vi "Main.vi"(1 "重新开始？":bool) -> ()   [LabVIEW 2018]
panel:
  out "时间标识":timestamp format="%<%H:%M:%S\n%x>T"
  in  "参数设置":bool=TRUE
  in  "退出":bool
  in  "读取历史数据":bool=TRUE
  in  "保存数据":bool=TRUE
  in  "开始测量":bool=TRUE
  out "实时消息":T1
  # "任务选择"
  # "开始测量"
  # "退 出"
  # "保存数据"
  # "读取历史数据"
  # "功率"
  # "能量"
  # "时间"
  # "光谱"
  # "偏振"
  # "近远场"
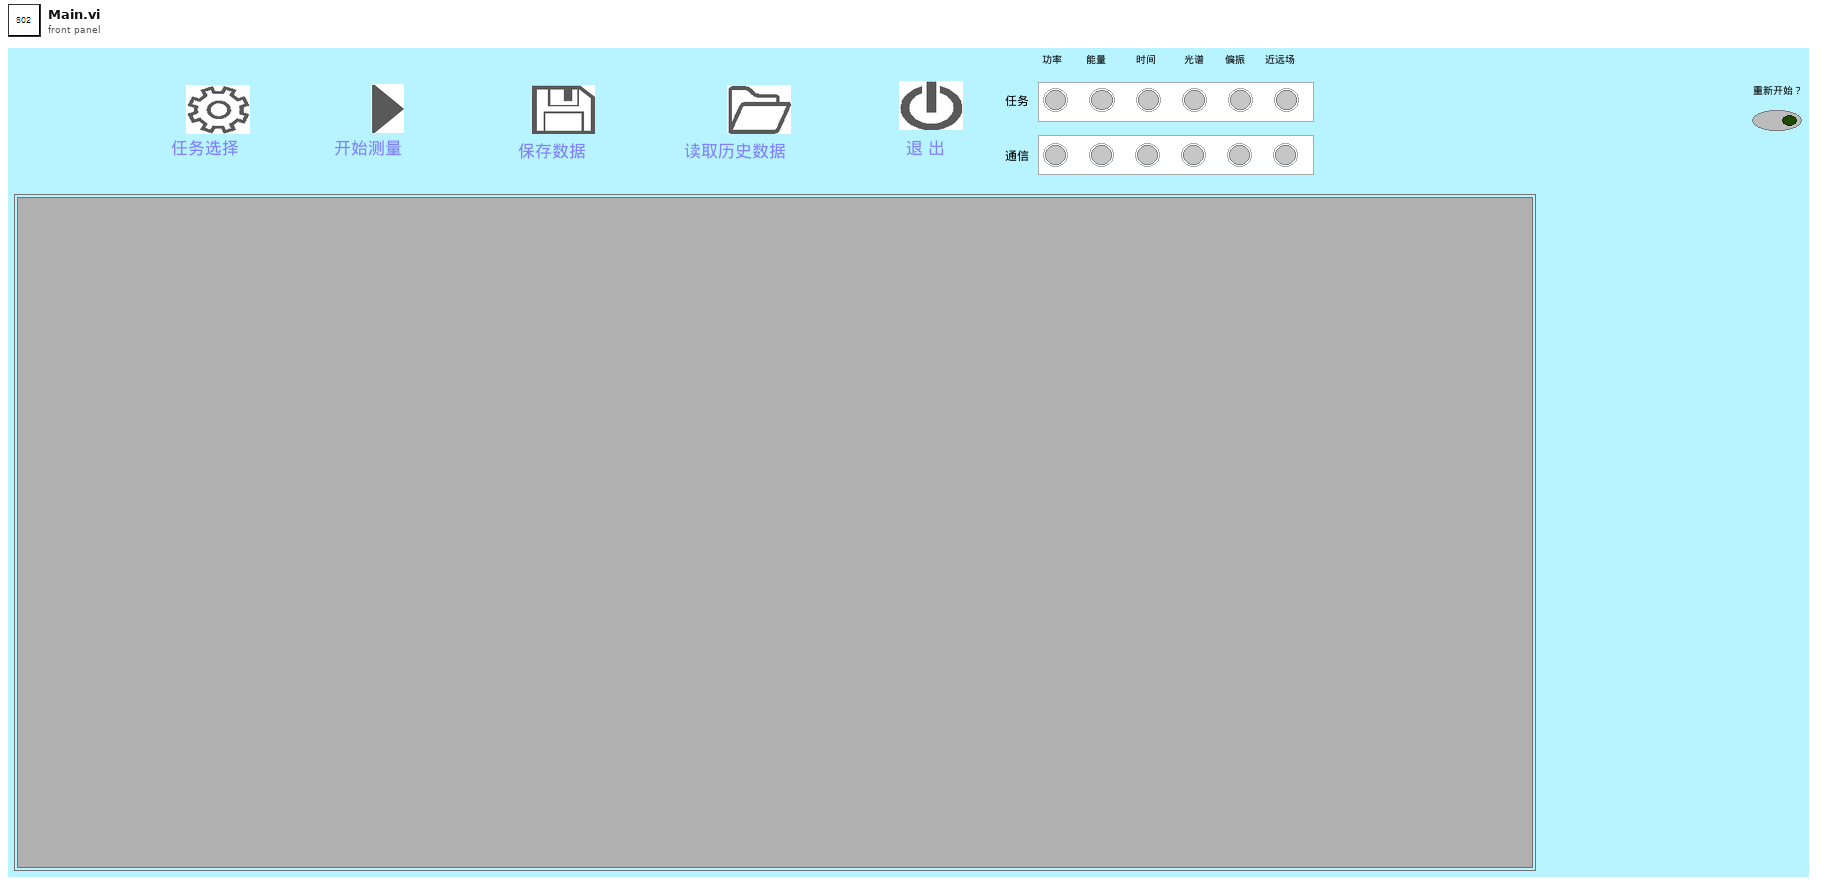
[diagram p1: front panel]
types:
  T1 = cluster{"任务":cluster{"功率任务":bool, "能量任务":bool, "时间波形任务":bool, "光谱任务":bool, "偏振任务":bool, "近远场任务":bool}, "通信":cluster{"功率通信":bool, "能量通信":bool, "时间波形通信":bool, "光谱通信":bool, "偏振通信":bool, "近远场通信":bool}}
  T2 = enum8{"Enabled", "Disabled", "Disabled and Grayed Out"}
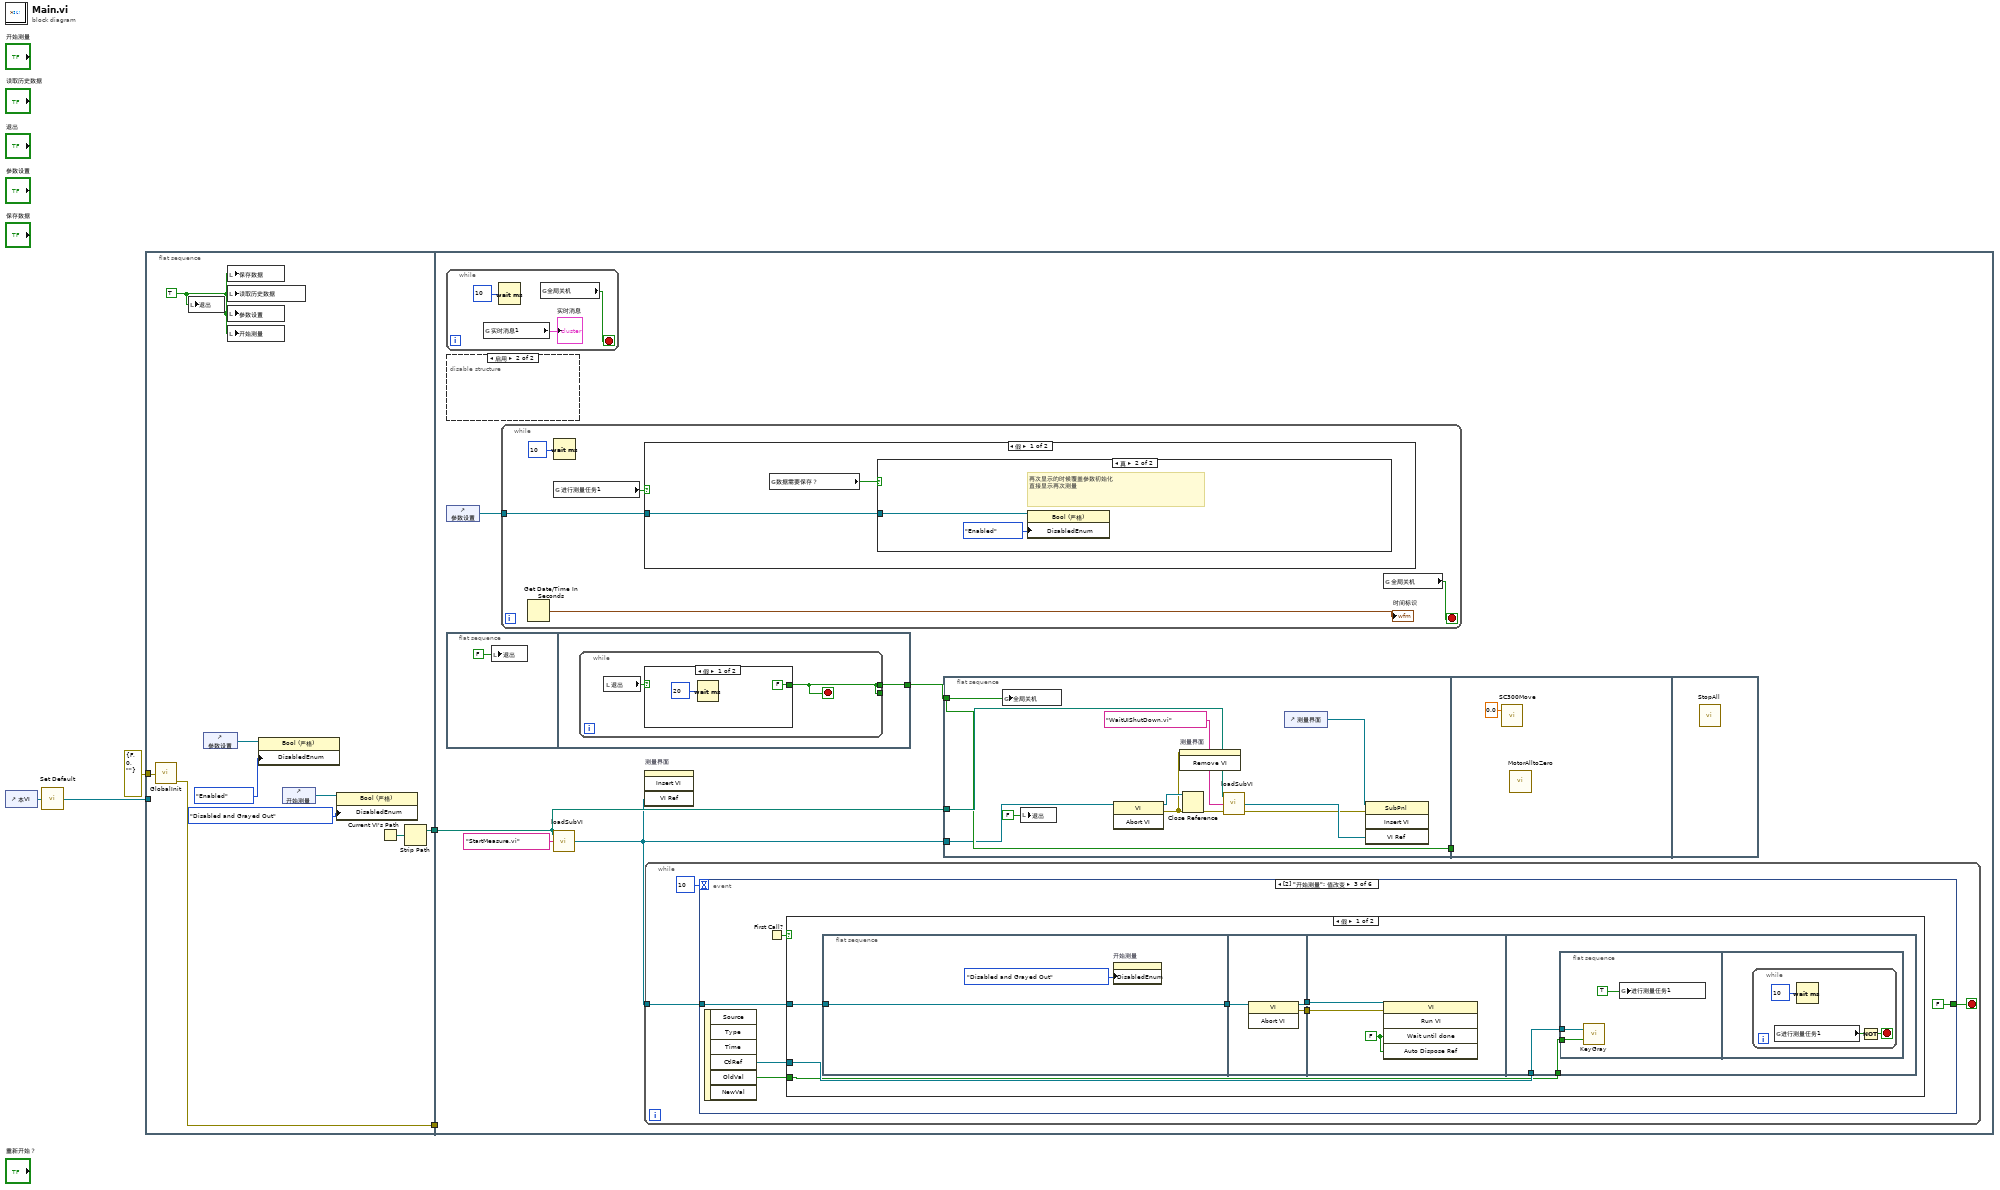
[diagram p0: block diagram]
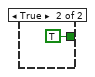
[diagram p2: hidden frame]
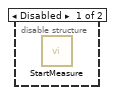
[diagram p3: hidden frame]
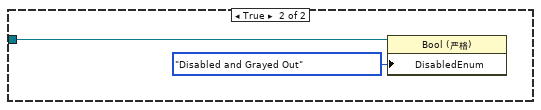
[diagram p5: hidden frame]
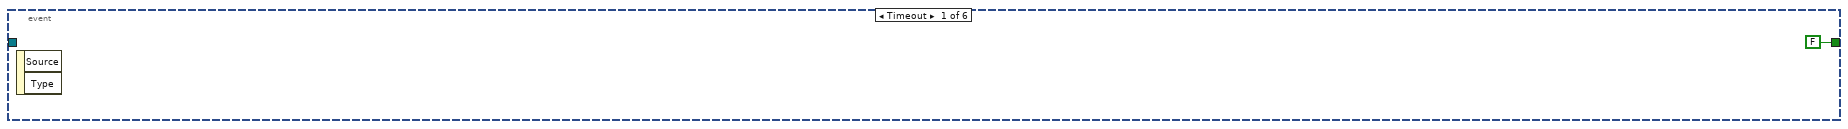
[diagram p6: hidden frame]
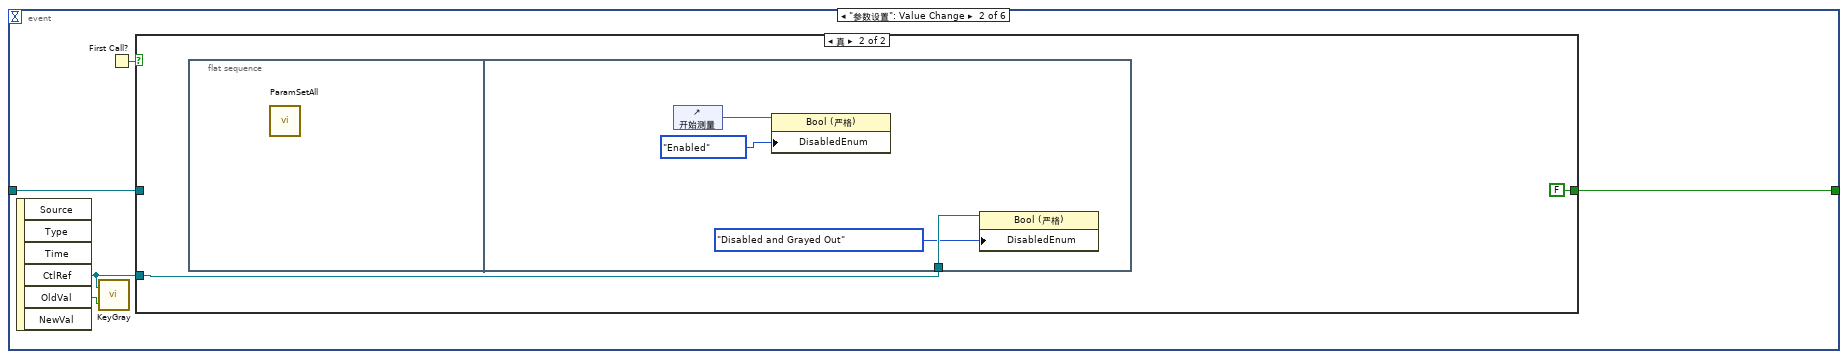
[diagram p7: hidden frame]
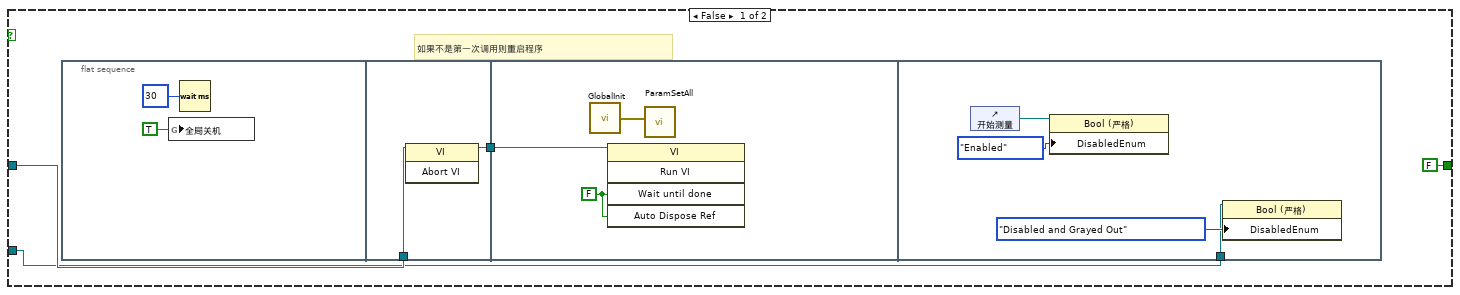
[diagram p8: hidden frame]
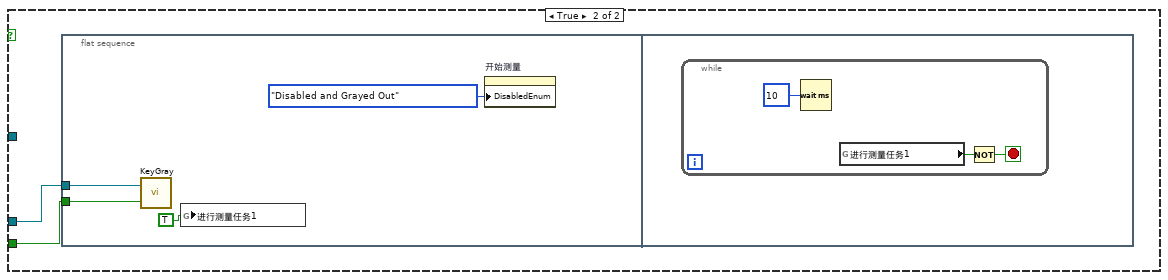
[diagram p9: hidden frame]
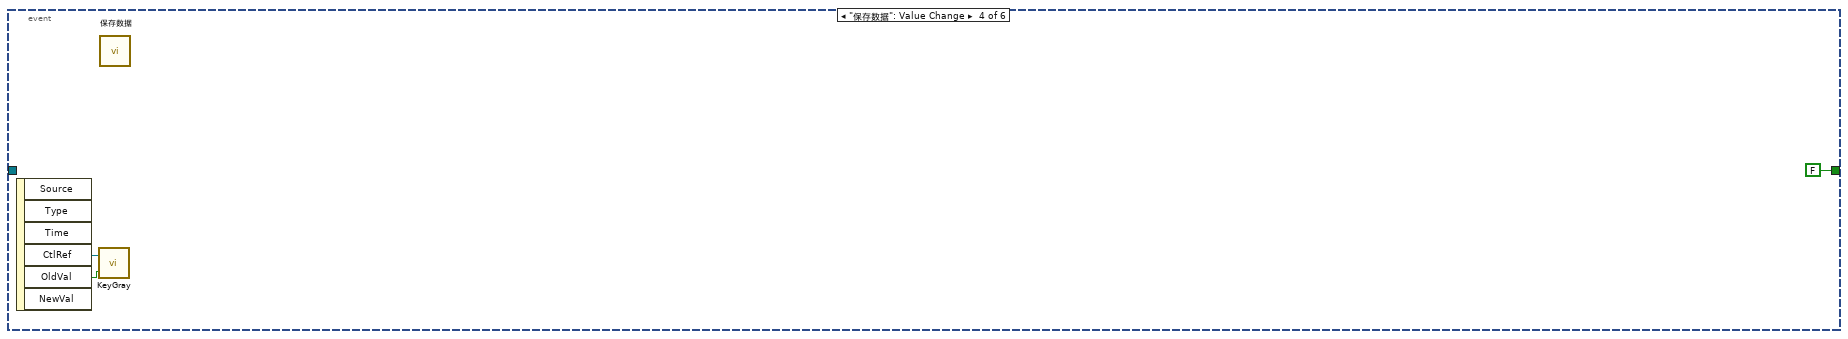
[diagram p10: hidden frame]
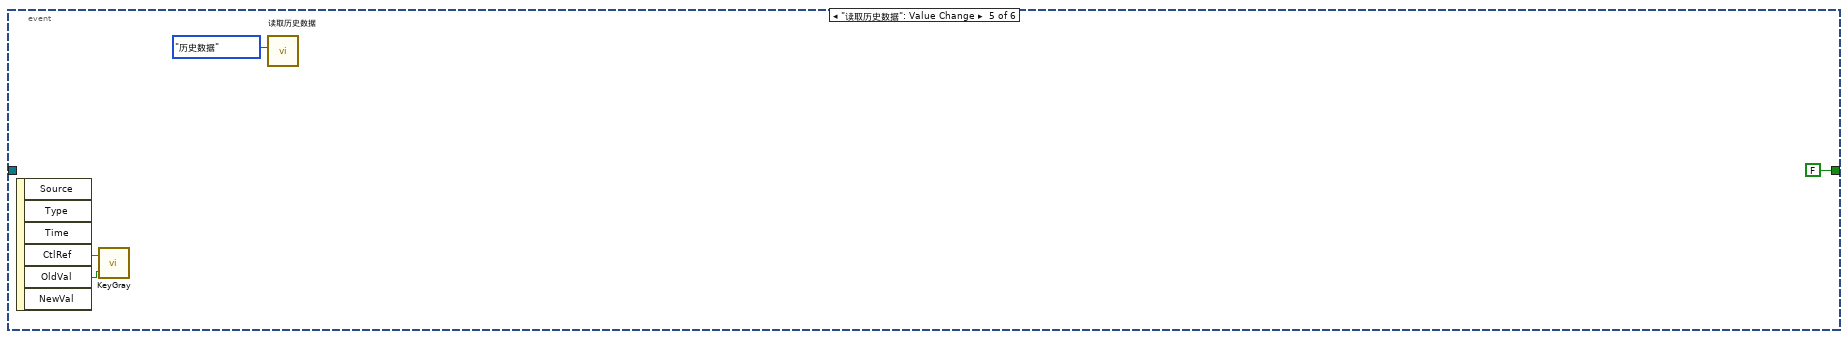
[diagram p11: hidden frame]
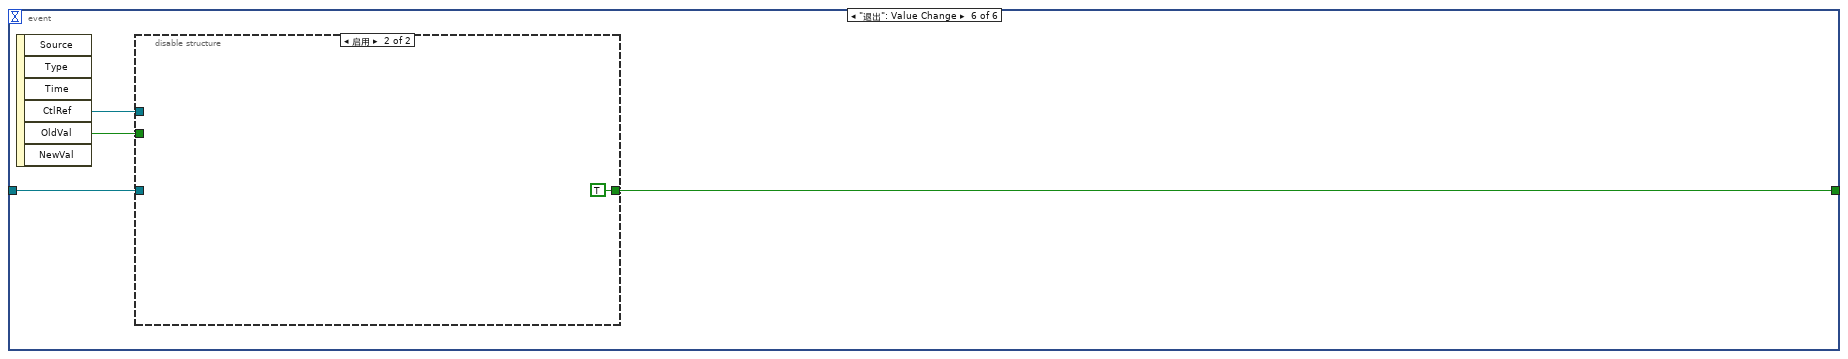
[diagram p12: hidden frame]
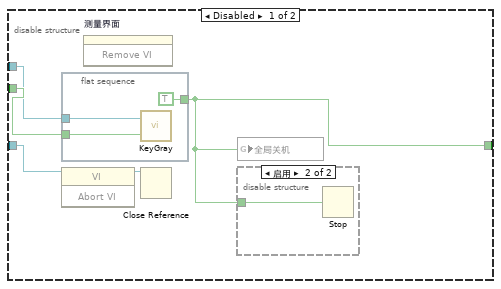
[diagram p13: hidden frame]
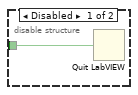
[diagram p14: hidden frame]
diagram:
  n1 = control-ref of="本VI"() -> (w3:refnum<vi>)
  n2 = call "Set Default.vi"("VI引用"=w3) -> ("引用输出"=w2:refnum<vi>)
  n3 = flat-sequence {
    tunnel: errorcluster {"status"=FALSE, "code"=0, "source"=""} ("错误输入（无错误）") -> [w13]
    tunnel: [w12] -> w4
    tunnel: w2 -> [_]
    tunnel: [w6] -> w1
    tunnel: w4 -> [_]
    tunnel: w1 -> [w16]
    frame #0 {
      w14 = TRUE
      n4 = call "GlobalInit.vi"("错误输入（无错误）"=w13) -> ("错误输出"=w12:errorcluster)
      n5 = local write "退出"(w14) -> ()
      n6 = control-ref of="参数设置"() -> (w11:refnum<vi>)
      n7 = local write "保存数据"(w14) -> ()
      n8 = local write "读取历史数据"(w14) -> ()
      n9 = local write "参数设置"(w14) -> ()
      n10 = local write "开始测量"(w14) -> ()
      n11 = property class="Bool (严格)"(reference=w11, "DisabledEnum"=T2."Enabled" ("禁用")) -> ()  [unwired: 1 in, 2 out]
      n12 = control-ref of="开始测量"() -> (w9:refnum<vi>)
      n13 = property class="Bool (严格)"(reference=w9, "DisabledEnum"=T2."Disabled and Grayed Out" ("禁用")) -> ()  [unwired: 1 in, 2 out]
      n14 = Current VI's Path() -> (path=w7:path)
      n15 = Strip Path(path=w7) -> (stripped path=w6:path)  [unwired: 1 out]
    }
    frame #1 {
      n16 = while {
        stop <- w52 stop-if-true
        n17 = global read "globalMessage.vi" "实时消息1"() -> (→"实时消息":T1)
        n18 = Wait (ms)(milliseconds to wait=u32 10 ("等待时间（毫秒）")) -> ()  [unwired: 1 out]
        n19 = global read "参数.vi" "全局关机"() -> (w52:bool)
      }
      n20 = disable-structure shown="启用" {
        frame Disabled {
          n21 = call "StartMeasure.vi"() -> ()  [unwired: 1 in, 1 out]
        }
        frame Enabled {
        }
      }
      n22 = control-ref of="参数设置"() -> (w20:refnum<vi>)
      n23 = flat-sequence {
        tunnel: [w22] -> w18
        frame #0 {
          n24 = local write "退出"(FALSE ("退出")) -> ()
        }
        frame #1 {
          n25 = while {
            tunnel: [w23] -> w22
            tunnel: [w23] -> _
            stop <- w23 stop-if-true
            n26 = local read "退出"() -> (w24:bool)
            n27 = case shown="假" w24 {
              tunnel: [FALSE TRUE] -> w23
              frame False {
                n28 = Wait (ms)(milliseconds to wait=u32 20 ("等待时间（毫秒）")) -> ()  [unwired: 1 out]
              }
              frame True {
              }
            }
          }
        }
      }
      n29 = while {
        tunnel: w20 -> [w43]
        stop <- w42 stop-if-true
        n30 = Get Date/Time In Seconds() -> (seconds since 1Jan1904=→"时间标识":timestamp)
        n31 = Wait (ms)(milliseconds to wait=u32 10 ("等待时间（毫秒）")) -> ()  [unwired: 1 out]
        n32 = global read "参数.vi" "进行测量任务1"() -> (w44:bool)
        n33 = case shown="假" w44 {
          tunnel: w43 -> [w46 w49]
          frame False {
            n34 = global read "globalMessage.vi" "数据需要保存？"() -> (w45:bool)
            n35 = case shown="真" w45 {
              tunnel: w46 -> [_ w47]
              frame False {
              }
              frame True {
                # "再次显示的时候覆盖参数初始化\n直接显示再次测量"
                n36 = property class="Bool (严格)"(reference=w47, "DisabledEnum"=T2."Enabled" ("禁用")) -> ()  [unwired: 1 in, 2 out]
              }
            }
          }
          frame True {
            n37 = property class="Bool (严格)"(reference=w49, "DisabledEnum"=T2."Disabled and Grayed Out" ("禁用")) -> ()  [unwired: 1 in, 2 out]
          }
        }
        n38 = global read "参数.vi" "全局关机"() -> (w42:bool)
      }
      n39 = call "loadSubVI.vi"("VI名称"="StartMeasure.vi", "基路径"=w16) -> ("SubVIRef"=w15:refnum<vi>)  [unwired: 2 in, 1 out]
      n40 = invoke on="测量界面" class="SubPnl" method="Insert VI"("VI Ref"=w15) -> ()  [unwired: 3 in, 4 out]
      n41 = while {
        tunnel: w15 -> [w54]
        stop <- w56 stop-if-true
        n42 = event shown="[2] \"开始测量\": 值改变" {
          selector: _ -> [_ _ _ _ _ _]
          dyn-events: _ -> [_ _ _ _ _ _]
          timeout: 10 -> [_ _ _ _ _ _]
          tunnel: [FALSE w59 FALSE FALSE FALSE w128] -> w56
          tunnel: w54 -> [_ w58 w84 _ _ w127]
          event Timeout {
            n43 = event-data() -> ()  [unwired: 1 in, 2 out]
          }
          event "参数设置": Value Change {
            n44 = event-data() -> ("CtlRef"=w61:refnum<vi>, "OldVal"=w62:bool)  [unwired: 1 in, 4 out]
            n45 = call "KeyGray.vi"("OldVal"=w62, "CtlRef"=w61) -> ()  [unwired: 1 in]
            n46 = First Call?() -> (First Call?: T/F=w60:bool)
            n47 = case shown="真" w60 {
              tunnel: w61 -> [w64 w79]
              tunnel: [FALSE FALSE] -> w59
              tunnel: w58 -> [w65 _]
              frame False {
                # "如果不是第一次调用则重启程序"
                n48 = flat-sequence {
                  tunnel: w65 -> [w70]
                  tunnel: [w69] -> w63
                  tunnel: w63 -> [w71]
                  tunnel: w64 -> [w74]
                  frame #0 {
                    n49 = global write "参数.vi" "全局关机"(TRUE ("全局关机")) -> ()
                    n50 = Wait (ms)(milliseconds to wait=u32 30 ("等待时间（毫秒）")) -> ()  [unwired: 1 out]
                  }
                  frame #1 {
                    n51 = invoke class="VI" method="Abort VI"(reference=w70) -> (reference out=w69:refnum<vi>)  [unwired: 2 in, 2 out]
                  }
                  frame #2 {
                    w72 = FALSE ("结束前等待")
                    n52 = call "GlobalInit.vi"() -> ("错误输出"=w73:errorcluster)  [unwired: 1 in]
                    n53 = invoke class="VI" method="Run VI"(reference=w71, "Wait until done"=w72, "Auto Dispose Ref"=w72) -> ()  [unwired: 2 in, 5 out]
                    n54 = call "ParamSetAll.vi"("error in (no error)"=w73) -> ()  [unwired: 11 in]
                  }
                  frame #3 {
                    n55 = control-ref of="开始测量"() -> (w77:refnum<vi>)
                    n56 = property class="Bool (严格)"(reference=w77, "DisabledEnum"=T2."Enabled" ("禁用")) -> ()  [unwired: 1 in, 2 out]
                    n57 = property class="Bool (严格)"(reference=w74, "DisabledEnum"=T2."Disabled and Grayed Out" ("禁用")) -> ()  [unwired: 1 in, 2 out]
                  }
                }
              }
              frame True {
                n58 = flat-sequence {
                  tunnel: w79 -> [w83]
                  frame #0 {
                    n59 = call "ParamSetAll.vi"() -> ()  [unwired: 12 in]
                  }
                  frame #1 {
                    n60 = control-ref of="开始测量"() -> (w81:refnum<vi>)
                    n61 = property class="Bool (严格)"(reference=w81, "DisabledEnum"=T2."Enabled" ("禁用")) -> ()  [unwired: 1 in, 2 out]
                    n62 = property class="Bool (严格)"(reference=w83, "DisabledEnum"=T2."Disabled and Grayed Out" ("禁用")) -> ()  [unwired: 1 in, 2 out]
                  }
                }
              }
            }
          }
          event "开始测量": Value Change {
            n63 = event-data() -> ("CtlRef"=w87:refnum<vi>, "OldVal"=w88:bool)  [unwired: 1 in, 4 out]
            n64 = First Call?() -> (First Call?: T/F=w85:bool)
            n65 = case shown="假" w85 {
              tunnel: w88 -> [w90 w112]
              tunnel: w87 -> [w91 w111]
              tunnel: w84 -> [w94 _]
              frame False {
                n66 = flat-sequence {
                  tunnel: w94 -> [w96]
                  tunnel: [w96] -> w89
                  tunnel: [w98] -> w93
                  tunnel: [w97] -> w92
                  tunnel: w89 -> [w99]
                  tunnel: w93 -> [w102]
                  tunnel: w92 -> [w101]
                  tunnel: w91 -> [w104]
                  tunnel: w90 -> [w103]
                  frame #0 {
                    n67 = property on="开始测量" class="Bool (严格)"("DisabledEnum"=T2."Disabled and Grayed Out" ("禁用")) -> ()  [unwired: 2 in, 2 out]
                  }
                  frame #1 {
                    n68 = invoke class="VI" method="Abort VI"(reference=w99) -> (reference out=w98:refnum<vi>, error out=w97:errorcluster)  [unwired: 2 in, 1 out]
                  }
                  frame #2 {
                    w100 = FALSE
                    n69 = invoke class="VI" method="Run VI"(reference=w102, error in=w101, "Wait until done"=w100, "Auto Dispose Ref"=w100) -> ()  [unwired: 1 in, 5 out]
                  }
                  frame #3 {
                    n70 = flat-sequence {
                      tunnel: w104 -> [w106]
                      tunnel: w103 -> [w105]
                      frame #0 {
                        n71 = call "KeyGray.vi"("OldVal"=w105, "CtlRef"=w106) -> ()  [unwired: 1 in]
                        n72 = global write "参数.vi" "进行测量任务1"(TRUE ("进行测量任务")) -> ()
                      }
                      frame #1 {
                        n73 = while {
                          stop <- w109 stop-if-true
                          n74 = global read "参数.vi" "进行测量任务1"() -> (w110:bool)
                          n75 = Wait (ms)(milliseconds to wait=u32 10 ("等待时间（毫秒）")) -> ()  [unwired: 1 out]
                          n76 = Not(x=w110) -> (.not. x?=w109:bool)
                        }
                      }
                    }
                  }
                }
              }
              frame True {
                n77 = flat-sequence {
                  tunnel: w112 -> [w115]
                  tunnel: w111 -> [w114]
                  frame #0 {
                    n78 = call "KeyGray.vi"("OldVal"=w115, "CtlRef"=w114) -> ()  [unwired: 1 in]
                    n79 = global write "参数.vi" "进行测量任务1"(TRUE ("进行测量任务")) -> ()
                    n80 = property on="开始测量" class="Bool (严格)"("DisabledEnum"=T2."Disabled and Grayed Out" ("禁用")) -> ()  [unwired: 2 in, 2 out]
                  }
                  frame #1 {
                    n81 = while {
                      stop <- w118 stop-if-true
                      n82 = Wait (ms)(milliseconds to wait=u32 10 ("等待时间（毫秒）")) -> ()  [unwired: 1 out]
                      n83 = global read "参数.vi" "进行测量任务1"() -> (w119:bool)
                      n84 = Not(x=w119) -> (.not. x?=w118:bool)
                    }
                  }
                }
              }
            }
          }
          event "保存数据": Value Change {
            n85 = event-data() -> ("CtlRef"=w122:refnum<vi>, "OldVal"=w121:bool)  [unwired: 1 in, 4 out]
            n86 = call "KeyGray.vi"("OldVal"=w121, "CtlRef"=w122) -> ()  [unwired: 1 in]
            n87 = call "保存数据.vi"() -> ()  [unwired: 12 in]
          }
          event "读取历史数据": Value Change {
            n88 = event-data() -> ("CtlRef"=w126:refnum<vi>, "OldVal"=w125:bool)  [unwired: 1 in, 4 out]
            n89 = call "KeyGray.vi"("OldVal"=w125, "CtlRef"=w126) -> ()  [unwired: 1 in]
            n90 = call "读取历史数据.vi"("进入状态"=enum16{"历史数据", "当前数据"}."历史数据") -> ()  [unwired: 11 in]
          }
          event "退出": Value Change {
            n91 = event-data() -> ("CtlRef"=w129:refnum<vi>, "OldVal"=w130:bool)  [unwired: 1 in, 4 out]
            n92 = disable-structure shown="启用" {
              disable-tunnel: w130 -> [w135 _]
              disable-tunnel: w129 -> [w134 _]
              disable-tunnel: [w133 TRUE] -> w128
              disable-tunnel: w127 -> [w131 _]
              frame Disabled {
                n93 = flat-sequence {
                  tunnel: w135 -> [w138]
                  tunnel: w134 -> [w137]
                  tunnel: [TRUE] -> w133
                  frame #0 {
                    n94 = call "KeyGray.vi"("OldVal"=w138, "CtlRef"=w137) -> ()  [unwired: 1 in]
                  }
                }
                n95 = invoke class="VI" method="Abort VI"(reference=w131) -> (reference out=w132:refnum<vi>)  [unwired: 2 in, 2 out]
                n96 = invoke on="测量界面" class="SubPnl" method="Remove VI"() -> ()  [unwired: 3 in, 3 out]
                n97 = Close Reference(reference=w132) -> ()  [unwired: 1 in, 1 out]
                n98 = global write "参数.vi" "全局关机"(w133) -> ()
                n99 = disable-structure shown="启用" {
                  disable-tunnel: w133 -> [w139 w140]
                  frame Disabled {
                    n100 = Quit LabVIEW(quit? (T)=w139) -> ()
                  }
                  frame Enabled {
                    n101 = Stop(stop? (T)=w140) -> ()
                  }
                }
              }
              frame Enabled {
              }
            }
          }
        }
      }
      n102 = flat-sequence {
        tunnel: w18 -> [w35]
        tunnel: [w35] -> w17
        tunnel: w16 -> [w38]
        tunnel: w15 -> [w31]
        tunnel: w17 -> [_]
        frame #0 {
          n103 = global write "参数.vi" "全局关机"(w35) -> ()
          n104 = local write "退出"(FALSE ("退出")) -> ()
          n105 = invoke class="VI" method="Abort VI"(reference=w31) -> (reference out=w32:refnum<vi>, error out=w30:errorcluster)  [unwired: 2 in, 1 out]
          n106 = invoke on="测量界面" class="SubPnl" method="Remove VI"(error in=w30) -> ()  [unwired: 2 in, 3 out]
          n107 = Close Reference(reference=w32, error in (no error)=w30) -> (error out=w29:errorcluster)
          n108 = call "loadSubVI.vi"("错误输入（无错误）"=w29, "VI名称"="WaitUIShutDown.vi", "基路径"=w38) -> ("错误输出"=w28:errorcluster, "SubVIRef"=w34:refnum<vi>)  [unwired: 1 in]
          n109 = control-ref of="测量界面"() -> (w36:refnum<vi>)
          n110 = invoke on="调用节点" class="SubPnl" method="Insert VI"(reference=w36, error in=w28, "VI Ref"=w34) -> ()  [unwired: 1 in, 4 out]
        }
        frame #1 {
          n111 = call "SC300Move.vi"("位置/mm"=0.0) -> ()  [unwired: 2 in, 1 out]
          n112 = call "MotorAlltoZero.vi"() -> ()  [unwired: 12 in]
        }
        frame #2 {
          n113 = call "StopAll.vi"() -> ()  [unwired: 12 in]
        }
      }
    }
  }
